vi "Chroma 1905x Series Configure DC CHK.vi"(8 "error in (no error)":errorcluster, 9 "CHK value":u8 max=1 step=1 format="%.0p", 10 "Step":T1=1 min=1 max=99 step=1, 11 "VISA resource name":refnum<visa-resource-name>) -> (0 "error out":errorcluster, 3 "VISA resource name out":refnum<visa-resource-name>)   [LabVIEW 2025]
uses:
  Type Def/steps--numeric.ctl
panel:
  # "Configure CHK value"
  # "(for DC mode ONLY)"
  # "0=Off /1=On"
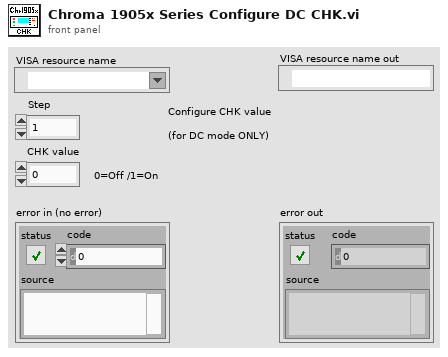
[diagram p1: front panel]
types:
  T1 = typedef "steps--numeric.ctl" = u8
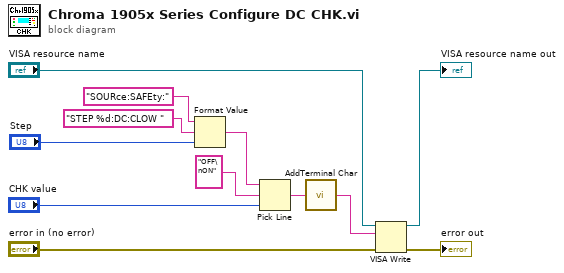
[diagram p0: block diagram]
diagram:
  n1 = Format Value(string ("")="SOURce:SAFEty:", format string="STEP %d:DC:CLOW ", value (0)="Step") -> (output string=w9:string)
  n2 = Pick Line(string ("")=w9, multi-line string="OFF\nON", line index="CHK value") -> (output string=w1:string)
  n3 = call "AddTerminal Char.vi"("Cmd string"=w1) -> ("Concatenated String"=w3:string)  [unwired: 4 in]
  n4 = VISA Write(VISA resource name="VISA resource name", write buffer=w3, error in (no error)="error in (no error)") -> (VISA resource name out=→"VISA resource name out":refnum<visa-resource-name>, error out=→"error out":errorcluster)  [unwired: 1 out]
